vi "on the relay numato.vi"() -> ()   [LabVIEW 2018]
panel:
  out "return count 6":u32
  in  "write buffer 3":string="relay readall\r\n"
  out "return count 5":u32
  out "read buffer 3":string
  out "return count 3":u32
  in  "write buffer 2":string="relay writeall ffffffff\r\n"
  out "return count 4":u32
  out "return count 2":u32
  out "return count":u32
  out "read buffer 2":string
  in  "error in (no error)":errorcluster
  out "error out":errorcluster
  in  "write buffer":string="relay readall\r\n"
  out "read buffer":string
  in  "VISA resource name":refnum<visa-resource-name>="TCPIP0::169.254.1.1::23::SOCKET"
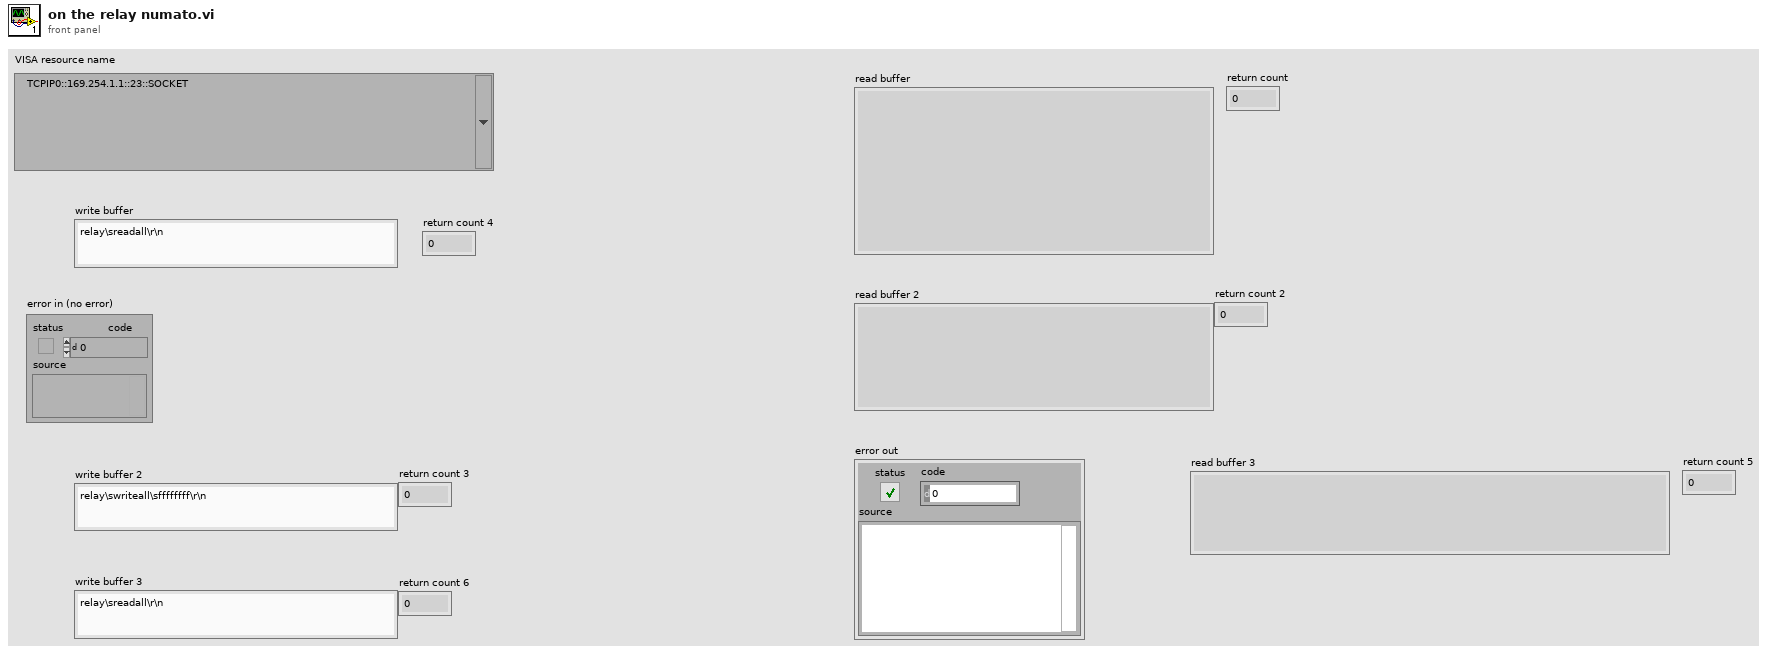
[diagram p1: front panel]
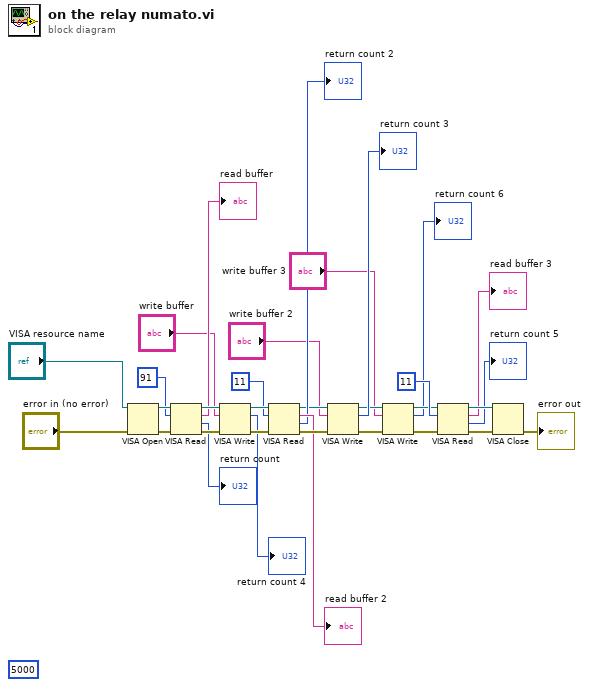
[diagram p0: block diagram]
diagram:
  (unwired) u32 5000 ("timeout (10sec)")
  n1 = VISA Open(error in (no error)="error in (no error)", VISA resource name="VISA resource name") -> (VISA resource name=w31:refnum<visa-resource-name>, error out=w30:errorcluster)  [unwired: 3 in]
  n2 = VISA Read(VISA resource name=w31, byte count=u32 91, error in (no error)=w30) -> (VISA resource name out=w28:refnum<visa-resource-name>, read buffer=→"read buffer":string, return count=→"return count":u32, error out=w27:errorcluster)
  n3 = VISA Write(VISA resource name=w28, write buffer="write buffer", error in (no error)=w27) -> (VISA resource name out=w24:refnum<visa-resource-name>, return count=→"return count 4":u32, error out=w23:errorcluster)
  n4 = VISA Read(VISA resource name=w24, byte count=u32 11, error in (no error)=w23) -> (VISA resource name out=w14:refnum<visa-resource-name>, read buffer=→"read buffer 2":string, return count=→"return count 2":u32, error out=w21:errorcluster)
  n5 = VISA Write(VISA resource name=w14, write buffer="write buffer 2", error in (no error)=w21) -> (VISA resource name out=w5:refnum<visa-resource-name>, return count=→"return count 3":u32, error out=w1:errorcluster)
  n6 = VISA Write(VISA resource name=w5, write buffer="write buffer 3", error in (no error)=w1) -> (VISA resource name out=w4:refnum<visa-resource-name>, return count=→"return count 6":u32, error out=w6:errorcluster)
  n7 = VISA Read(VISA resource name=w4, byte count=u32 11, error in (no error)=w6) -> (VISA resource name out=w10:refnum<visa-resource-name>, read buffer=→"read buffer 3":string, return count=→"return count 5":u32, error out=w11:errorcluster)
  n8 = VISA Close(VISA resource name=w10, error in (no error)=w11) -> (error out=→"error out":errorcluster)
